vi "Search Current.vi"(5 "BoardHandle in":T1, 7 "Channel # in":i32, 11 "error in (no error)":errorcluster, 12 "Stop Program Search Current":bool) -> (1 "Actual Voltage Level (V)":dbl format="%#_13g", 2 "Power Supply Trip":bool, 3 "Actual Current Limit (nA)":dbl format="%#_13g", 10 "Array":dbl[](array[numeric]), 14 "BoardHandle out 2":T1, 15 "error out":errorcluster)   [LabVIEW 2020]
uses:
  <instrlib>/CAEN PSM/CAEN PSM.lvlib
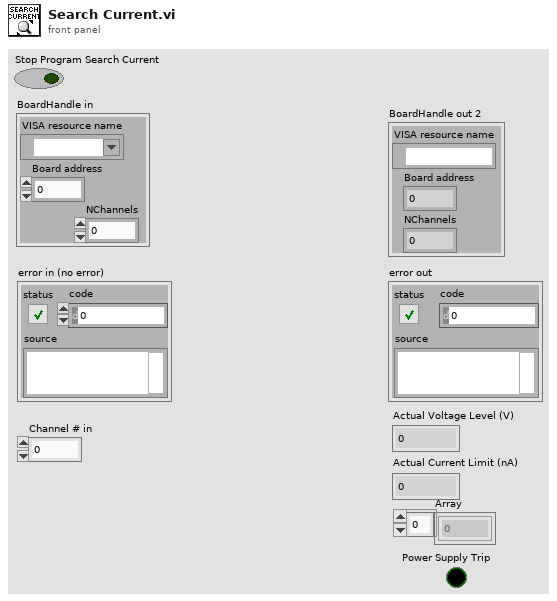
[diagram p1: front panel]
types:
  T1 = cluster{"VISA resource name":refnum<visa-resource-name>, "Board address":u8, "NChannels":u8}
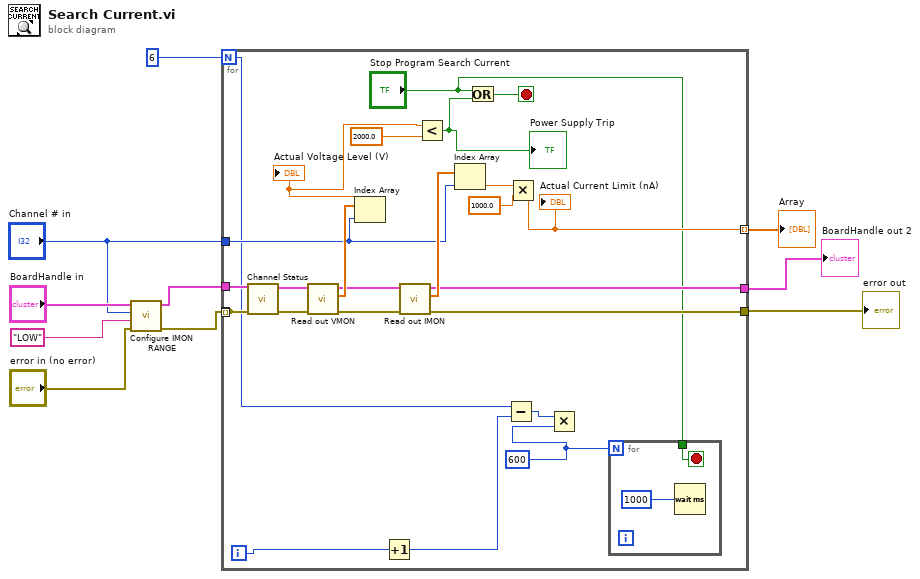
[diagram p0: block diagram]
diagram:
  n1 = call <instrlib>:"Configure IMON RANGE.vi"("error in (no error)"="error in (no error)", "IMon range (LOW)"="LOW", "Channel (0)"="Channel # in", "BoardHandle"="BoardHandle in") -> ("error out"=w4:errorcluster, "BoardHandle out"=w5:T1)  [unwired: 6 in]
  n2 = for {
    N: 6 ("N") -> [w20]
    tunnel: w4 -> [w25]
    tunnel: "Channel # in" -> [w26]
    tunnel: [w28] -> w8
    tunnel: [w27] -> w9
    tunnel: [w21] -> w10 mode=indexing
    tunnel: w5 -> [w24]
    tunnel: [w25] -> _ mode=indexing
    i -> [w18]
    stop <- w14 stop-if-true
    w12 = 600 ("dt (s) in")
    n3 = call <instrlib>:"Channel Status.vi"("error in (no error)"=w25, "BoardHandle"=w24) -> ("error out"=w34:errorcluster, "BoardHandle out"=w33:T1)  [unwired: 7 in, 1 out]
    n4 = call <instrlib>:"Read out VMON.vi"("error in (no error)"=w34, "BoardHandle"=w33) -> ("error out"=w30:errorcluster, "VMon values (V)"=w32:dbl[], "BoardHandle out"=w31:T1)  [unwired: 7 in]
    n5 = Index Array(array=w32, index=w26) -> (element=w16:dbl)
    "Actual Voltage Level (V)" <- w16
    n6 = Increment(x=w18) -> (x+1=w17:i32)
    n7 = call <instrlib>:"Read out IMON.vi"("error in (no error)"=w30, "BoardHandle"=w31) -> ("error out"=w27:errorcluster, "IMon values (uA)"=w29:dbl[], "BoardHandle out"=w28:T1)  [unwired: 6 in, 1 out]
    n8 = Less?(x=w16, y=2000.0) -> (x < y?=w13:bool)
    "Power Supply Trip" <- w13
    n9 = Index Array(array=w29, index=w26) -> (element=w23:dbl)
    n10 = Or(x="Stop Program Search Current", y=w13) -> (x .or. y?=w14:bool)
    n11 = Subtract(x=w20, y=w17) -> (x-y=w19:i32)
    n12 = Multiply(x=w23, y=1000.0) -> (x*y=w21:dbl)
    "Actual Current Limit (nA)" <- w21
    n13 = Multiply(x=w19, y=w12) -> ()  [unwired: 1 out]
    n14 = for {
      N: w12 -> [_]
      tunnel: "Stop Program Search Current" -> [w35]
      stop <- w35 stop-if-true
      n15 = Wait (ms)(milliseconds to wait=1000) -> ()  [unwired: 1 out]
    }
  }
  "Array" <- w10
  "error out" <- w9
  "BoardHandle out 2" <- w8
